vi "Simulate Gatling Gun.vi"(8 "error in (no error)":errorcluster, 11 "# of Measurements":i32=200) -> (0 "error out":errorcluster, 1 "Gun Trigger Time (ms)":u32=19055974, 2 "# of Triggers Sent":i32, 3 "Position vs Trigger":cluster{dbl[], dbl[]}[](graph))   [LabVIEW 2019]
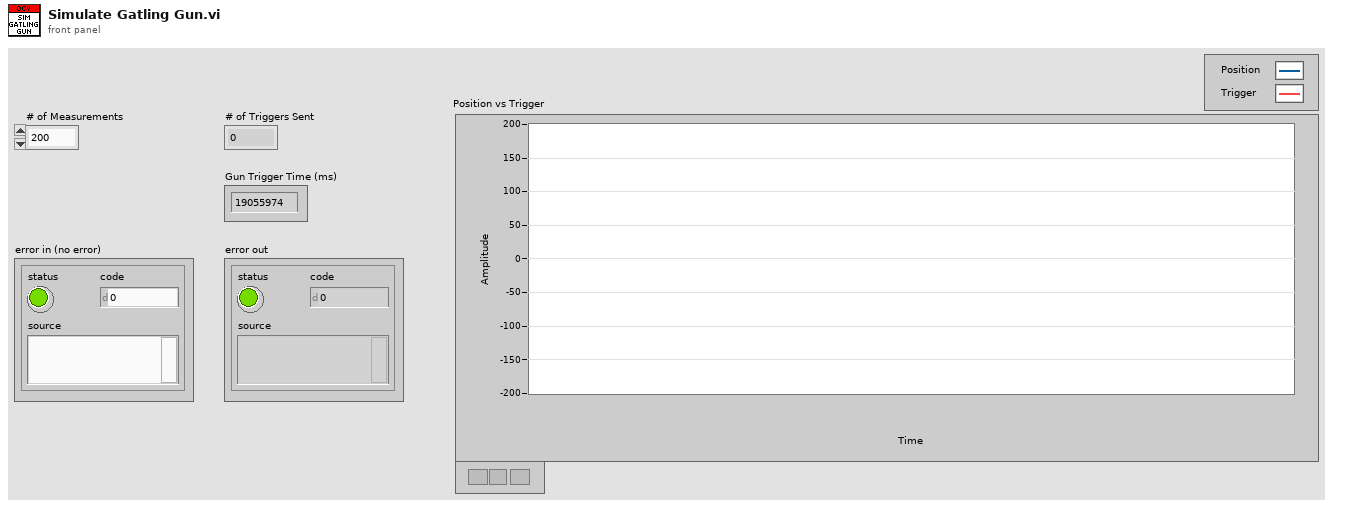
[diagram p1: front panel]
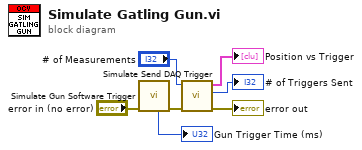
[diagram p0: block diagram]
diagram:
  n1 = call "Simulate Gun Software Trigger.vi"("error in (no error)"="error in (no error)") -> ("error out"=w4:errorcluster, "Gun Trigger Time (ms)"=→"Gun Trigger Time (ms)":u32)  [unwired: 9 in]
  n2 = call "Simulate Send DAQ Trigger.vi"("error in (no error)"=w4, "# of Triggers"="# of Measurements") -> ("error out"=→"error out":errorcluster, "# of Triggers Sent"=→"# of Triggers Sent":i32, "Position vs Trigger"=→"Position vs Trigger":cluster{dbl[], dbl[]}[])  [unwired: 7 in]
